vi "read_TCUStatus4_2.vi"(1 "Array":u8[](array[numeric])=[0, 0, 0, 0, 0, 0, 0, 0, 0, 0, 0, 0, 0, 0, 0, 0, 0, 0, 0, 0, 0, 0, 0, 0, 0, 0, 0, 0, 0, 0, 0, 0, 0, 0, 0, 0, 0, 0, 0, 0, 0, 0, 0, 0, 0, 0, 0, 0, 0, 0, 0, 0, 0, 0, 0, 0, 0, 0, 0, 0, 0, 0, 0, 0, 0, 0, 0, 0, 0, 0, 0, 0, 0, 0, 0, 0, 0, 0, 0, 0, 0, 0, 0, 0, 0, 0, 0, 0, 0, 0, 0, 0, 0, 0, 0, 0, 0, 0, 0, 0, 0, 0, 0, 0, 0, 0, 0, 0, 0, 0, 0, 0, 0, 0, 0, 0, 0, 0, 0, 0, 0, 0, 0, 0, 0, 0, 0, 0, 0, 0, 0, 0, 0, 0, 0, 0, 0, 0, 0, 0, 0, 0, 0, 0, 0, 0, 0, 0, 0, 0, 0, 0, 0, 0, 0, 0, 0, 0, 0, 0, 0, 0, 0, 0, 0, 0, 0, 0, 0, 0, 0, 0, 0, 0, 0, 0, 0, 0, 0, 0, 0]) -> (0 "Message":T1)   [LabVIEW 2017]
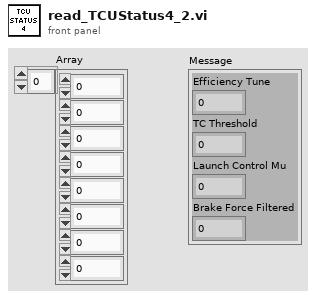
[diagram p1: front panel]
types:
  T1 = cluster{"Efficiency Tune":dbl, "TC Threshold":u8, "Launch Control Mu":dbl, "Brake Force Filtered":u16}
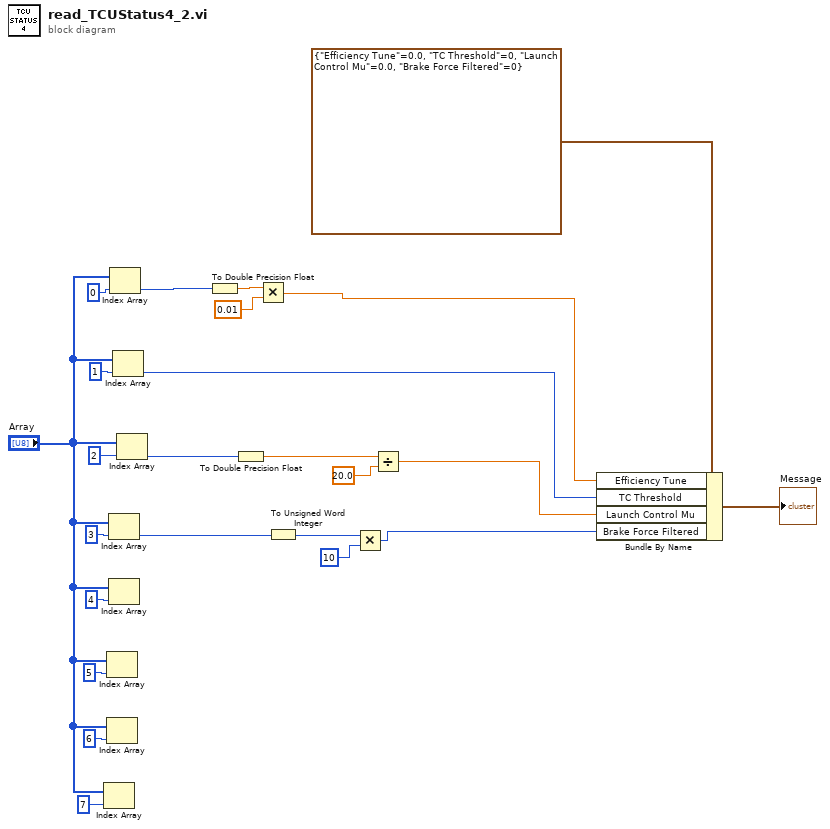
[diagram p0: block diagram]
diagram:
  n1 = Index Array(array="Array", index=7) -> ()  [unwired: 1 out]
  n2 = Index Array(array="Array", index=5) -> ()  [unwired: 1 out]
  n3 = Index Array(array="Array", index=6) -> ()  [unwired: 1 out]
  n4 = Index Array(array="Array", index=3) -> (element=w3:u8)
  n5 = Index Array(array="Array", index=4) -> ()  [unwired: 1 out]
  n6 = Index Array(array="Array", index=0) -> (element=w12:u8)
  n7 = Index Array(array="Array", index=1) -> (element=w7:u8)
  n8 = Index Array(array="Array", index=2) -> (element=w10:u8)
  n9 = To Double Precision Float(number=w12) -> (double precision float=w14:dbl)
  n10 = To Double Precision Float(number=w10) -> (double precision float=w6:dbl)
  n11 = Multiply(x=w14, y=0.01) -> (x*y=w8:dbl)
  n12 = To Unsigned Word Integer(number=w3) -> (unsigned 16bit integer=w5:u16)
  n13 = Multiply(x=w5, y=u16 10) -> (x*y=w2:u16)
  n14 = Divide(x=w6, y=20.0) -> (x/y=w9:dbl)
  n15 = Bundle By Name(cluster=T1 {"Efficiency Tune"=0.0, "TC Threshold"=0, "Launch Control Mu"=0.0, "Brake Force Filtered"=0}, "Efficiency Tune"=w8, "TC Threshold"=w7, "Launch Control Mu"=w9, "Brake Force Filtered"=w2) -> (→"Message":T1)
